vi "DO init.vi"(7 "N_moduls":i32, 10 "N_param":i32) -> (0 "error":errorcluster, 3 "DO":T1)   [LabVIEW 2019, in "Inputs.lvlib"]
uses:
  Inputs.lvlib
  Ctl/DO.ctl
  Ctl/Parameter State.ctl
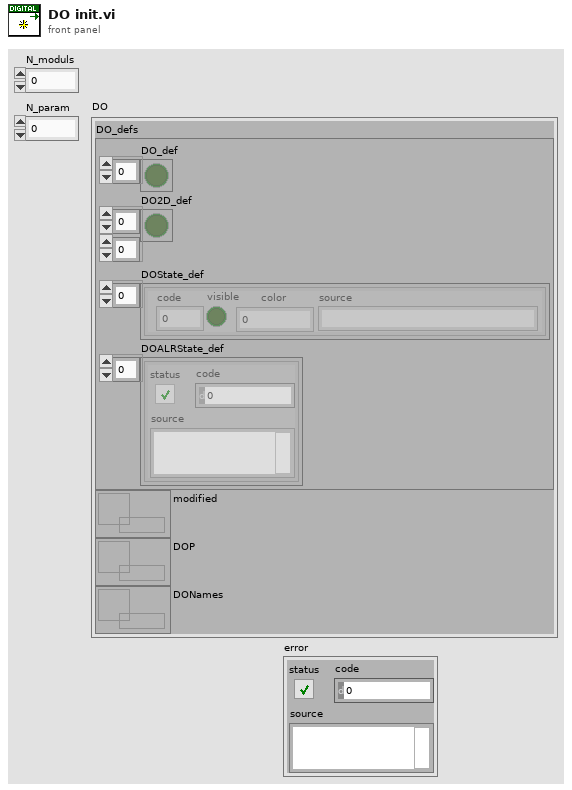
[diagram p1: front panel]
types:
  T1 = typedef "Inputs.lvlib/DO.ctl" = cluster{"DO_defs":cluster{"DO_def":bool[], "DO2D_def":bool[][], "DOState_def":T2[], "DOALRState_def":errorcluster[]}, "modified":refnum<data-value>, "DOP":refnum<data-value>, "DONames":refnum<data-value>}
  T2 = typedef "Inputs.lvlib/Parameter State.ctl" = cluster{"code":i32, "visible":bool, "color":u32, "source":string}
  T3 = cluster{"DO_def":bool[], "DO2D_def":bool[][], "DOState_def":T2[], "DOALRState_def":errorcluster[]}
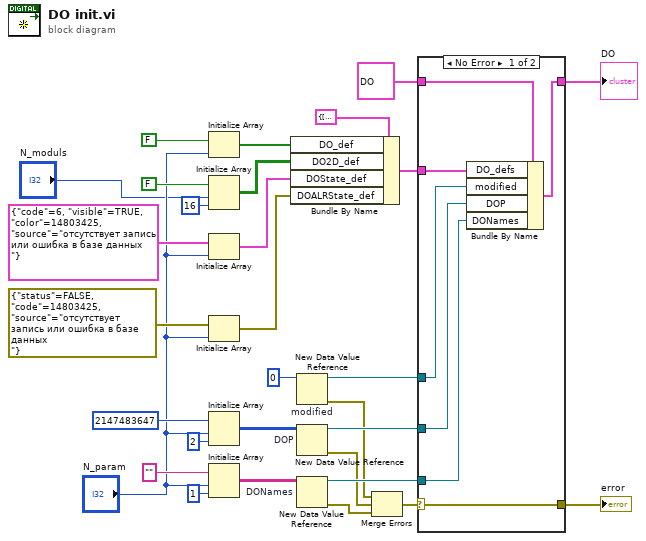
[diagram p0: block diagram]
diagram:
  n1 = Initialize Array(FALSE, "N_param") -> (w28:bool[])
  n2 = Initialize Array(FALSE, "N_moduls", 16 ("dimension size")) -> (w12:bool[][])
  n3 = Initialize Array(T2 {"code"=6, "visible"=TRUE, "color"=14803425, "source"="отсутствует запись или ошибка в базе данных                                                                                    "} ("STATE"), "N_param") -> (w13:T2[])
  n4 = Initialize Array(errorcluster {"status"=FALSE, "code"=14803425, "source"="отсутствует запись или ошибка в базе данных                                                                                    "} ("ALRSTATE"), "N_param") -> (w14:errorcluster[])
  n5 = Initialize Array(2147483647 ("DOP"), "N_param", 2 ("dimension size")) -> (w8:i32[][])
  n6 = Initialize Array("" ("AINames"), "N_param", 1 ("dimension size")) -> (w22:string[][])
  n7 = Bundle By Name(cluster=T3 {"DO_def"=[], "DO2D_def"=[], "DOState_def"=[], "DOALRState_def"=[]} ("DO_defs"), "DO_def"=w28, "DO2D_def"=w12, "DOState_def"=w13, "DOALRState_def"=w14) -> (w19:T3)
  n8 = New Data Value Reference "modified"(data value=u8 0 ("modified")) -> (data value reference=w6:refnum<data-value>, error out=w4:errorcluster)  [unwired: 1 in]
  n9 = New Data Value Reference "DOP"(data value=w8) -> (data value reference=w7:refnum<data-value>, error out=w3:errorcluster)  [unwired: 1 in]
  n10 = New Data Value Reference "DONames"(data value=w22) -> (data value reference=w21:refnum<data-value>, error out=w2:errorcluster)  [unwired: 1 in]
  n11 = Merge Errors(w4, w3, w2) -> (w5:errorcluster)
  n12 = case shown="No Error" w5 {
    selector: w5 -> [w34 w39]
    tunnel: w7 -> [w32 _]
    tunnel: w21 -> [w33 _]
    tunnel: [w34 w39] -> w20
    tunnel: w19 -> [w36 _]
    tunnel: T1 {"DO_defs"={"DO_def"=[], "DO2D_def"=[], "DOState_def"=[], "DOALRState_def"=[]}, "modified"=refnum, "DOP"=refnum, "DONames"=refnum} ("DO") -> [w37 w38]
    tunnel: [w35 w38] -> w17
    tunnel: w6 -> [w31 _]
    frame No Error {
      n13 = Bundle By Name(cluster=w37, "DO_defs"=w36, "modified"=w31, "DOP"=w32, "DONames"=w33) -> (w35:T1)
    }
    frame Error {
    }
  }
  "error" <- w20
  "DO" <- w17
